vi "74HC162.vi"(0 "EP":bool, 1 "D2":bool, 2 "D3":bool, 5 "ET":bool, 7 "cp":bool, 9 "CR`":bool, 11 "LD`":bool, 12 "D1":bool, 13 "D0":bool) -> (4 "Q3":bool, 6 "Q2":bool, 8 "Q1":bool, 10 "Q0":bool, 15 "RCO":bool)   [LabVIEW 2018]
panel:
  # "74HC162：十进制同步加法器"
  # "CR`：异步清零端\nEP：计数使能\nLD`：数据加载\nRC0：进位输出\nET：计数控制端"
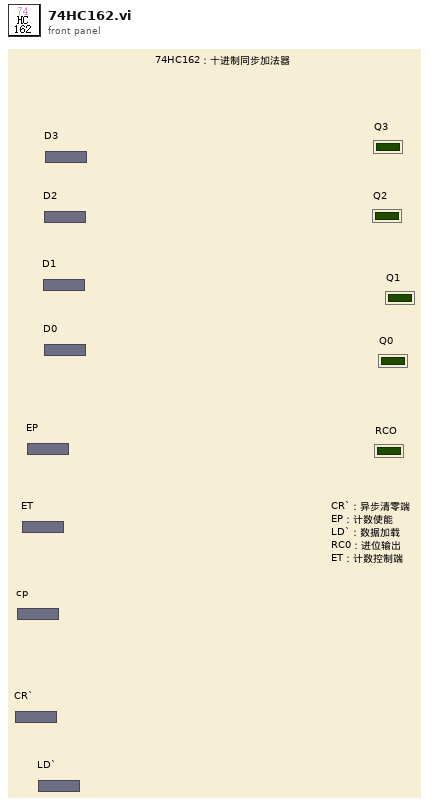
[diagram p1: front panel]
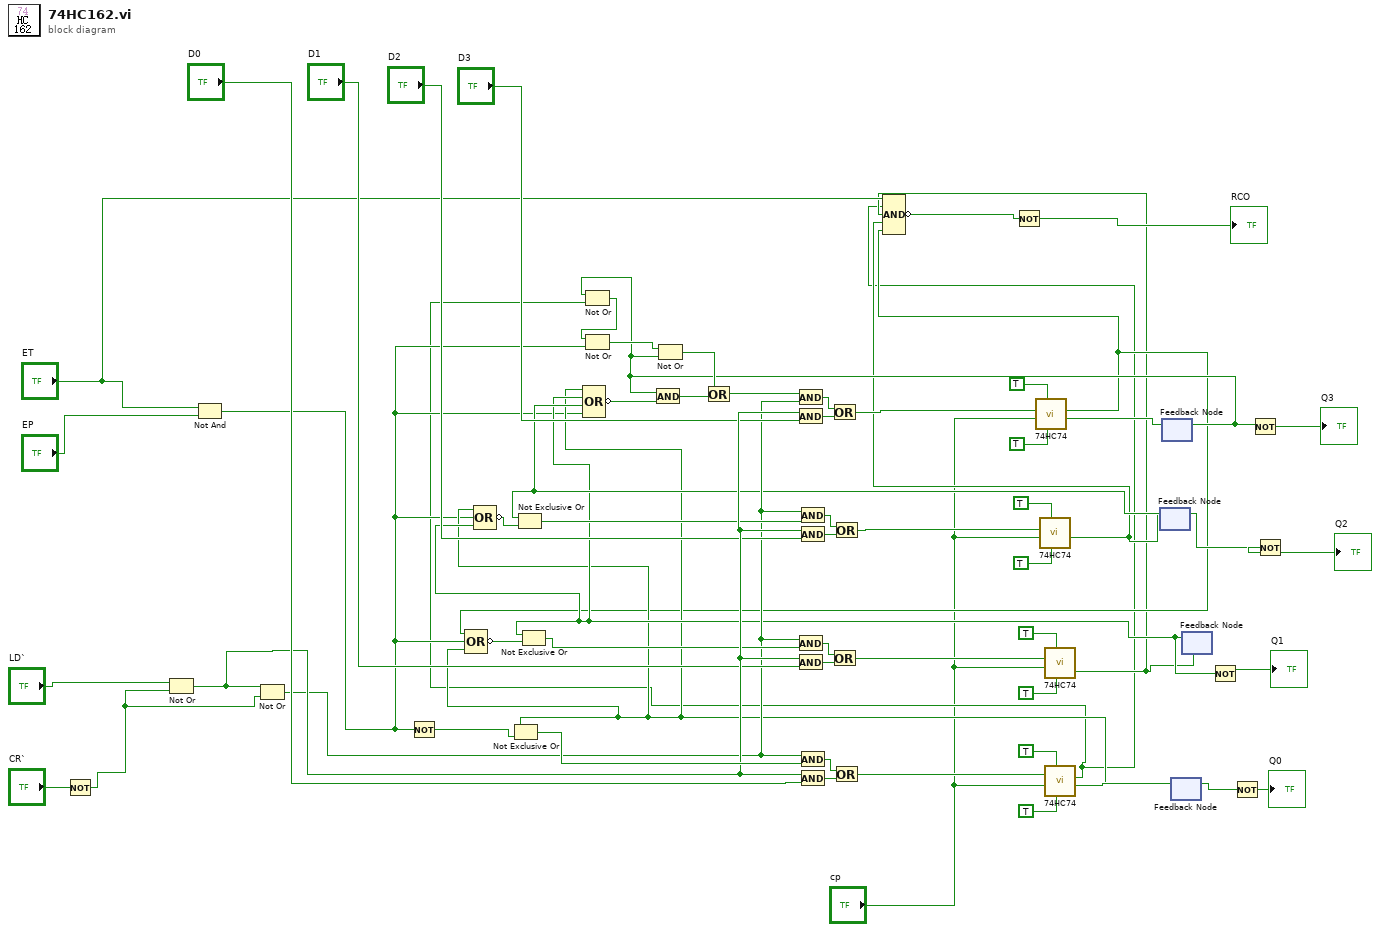
[diagram p0: block diagram]
diagram:
  n1 = Not(x="CR`") -> (.not. x?=w33:bool)
  n2 = Not Or(1:w33, 2:"LD`") -> (0:w29:bool)
  n3 = Not And(1:"EP", 2:"ET") -> (0:w10:bool)
  n4 = Not Or(1:w33, 2:w29) -> (0:w20:bool)
  n5 = Not(x=w10) -> (.not. x?=w30:bool)
  n6 = And(x=w29, y="D3") -> (x .and. y?=w41:bool)
  n7 = And(x=w29, y="D1") -> (x .and. y?=w45:bool)
  n8 = And(x=w29, y="D2") -> (x .and. y?=w43:bool)
  n9 = And(x=w29, y="D0") -> (x .and. y?=w47:bool)
  n10 = feedback #1() -> (w15:bool)  [unwired: 1 in]
  n11 = feedback #2() -> (w8:bool)  [unwired: 1 in]
  n12 = feedback #3() -> (w13:bool)  [unwired: 1 in]
  n13 = Not Exclusive Or(1:w30, 2:w13) -> (0:w31:bool)
  n14 = And(x=w20, y=w31) -> (x .and. y?=w48:bool)
  n15 = Or(x=w48, y=w47) -> (x .or. y?=w40:bool)
  n16 = call "74HC74.vi"("R`"=TRUE, "S`"=TRUE, "cp"="cp", "D"=w40) -> ("Q`"=w28:bool, "Q"=w3:bool)  [unwired: 6 in]
  n17 = Not Or(1:w3, 2:w8) -> (0:w9:bool)
  n18 = Not Or(1:w10, 2:w9) -> (0:w16:bool)
  n19 = Not Or(1:w8, 2:w16) -> (0:w17:bool)
  n20 = feedback-in #3(w28) -> ()
  n21 = feedback #4() -> (w14:bool)  [unwired: 1 in]
  n22 = Compound Arithmetic op=OR ("复合运算")(w13, w10, w14) -> (invert w21:bool)
  n23 = Not Exclusive Or(1:w21, 2:w15) -> (0:w23:bool)
  n24 = Compound Arithmetic op=OR ("复合运算")(w13, w14, w15, w10) -> (invert w12:bool)
  n25 = And(x=w8, y=w12) -> (x .and. y?=w18:bool)
  n26 = Or(x=w17, y=w18) -> (x .or. y?=w19:bool)
  n27 = And(x=w19, y=w20) -> (x .and. y?=w42:bool)
  n28 = And(x=w20, y=w23) -> (x .and. y?=w44:bool)
  n29 = Or(x=w42, y=w41) -> (x .or. y?=w37:bool)
  n30 = Or(x=w44, y=w43) -> (x .or. y?=w38:bool)
  n31 = call "74HC74.vi"("R`"=TRUE, "S`"=TRUE, "cp"="cp", "D"=w37) -> ("Q`"=w11:bool, "Q"=w7:bool)  [unwired: 6 in]
  n32 = Compound Arithmetic op=OR ("复合运算")(w7, w10, w13) -> (invert w22:bool)
  n33 = Not Exclusive Or(1:w22, 2:w14) -> (0:w24:bool)
  n34 = And(x=w20, y=w24) -> (x .and. y?=w46:bool)
  n35 = Or(x=w46, y=w45) -> (x .or. y?=w39:bool)
  n36 = call "74HC74.vi"("R`"=TRUE, "S`"=TRUE, "cp"="cp", "D"=w38) -> ("Q`"=w5:bool)  [unwired: 6 in, 1 out]
  n37 = call "74HC74.vi"("R`"=TRUE, "S`"=TRUE, "cp"="cp", "D"=w39) -> ("Q`"=w4:bool)  [unwired: 6 in, 1 out]
  n38 = Compound Arithmetic op=AND ("复合运算")("ET", w3, w4, w5, w7) -> (invert w2:bool)
  n39 = Not(x=w2) -> (.not. x?=→"RCO":bool)
  n40 = feedback-in #1(w5) -> ()
  n41 = feedback-in #2(w11) -> ()
  n42 = feedback-in #4(w4) -> ()
  n43 = Not(x=w14) -> (.not. x?=→"Q1":bool)
  n44 = Not(x=w13) -> (.not. x?=→"Q0":bool)
  n45 = Not(x=w8) -> (.not. x?=→"Q3":bool)
  n46 = Not(x=w15) -> (.not. x?=→"Q2":bool)
